vi "Untitled 4.vi"() -> ()   [LabVIEW 2017]
uses:
  <vilib>/Utility/NIReport.llb/Append Text Table to Report (wrap).vi
  <vilib>/Utility/NIReport.llb/NI_report.lvclass
panel:
  in  "Table Control":string[][](table)
  in  "template (empty)":path
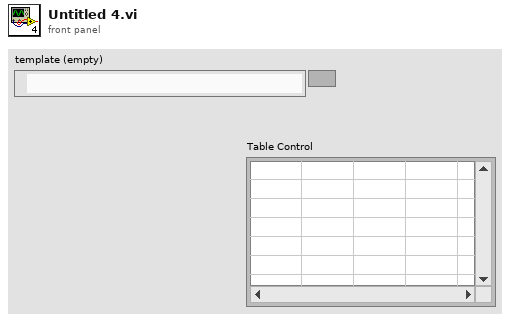
[diagram p1: front panel]
types:
  T1 = cluster{"position (excel)":cluster{"row":i32, "column":i32}, "name (excel)":string, "bookmark (word)":string}
  T2 = enum16{"maximized", "minimized", "normal", "no change"}
  T3 = enum16{"Standard Report", "HTML", "Word", "Excel"}
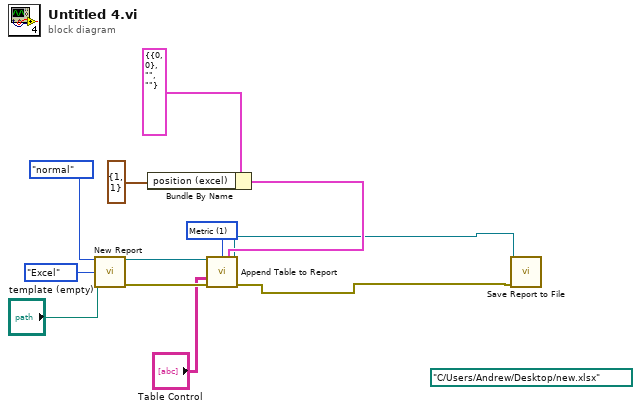
[diagram p0: block diagram]
diagram:
  (unwired) path "C:/Users/Andrew/Desktop/new.xlsx"
  w4 = u16 1 items=["US", "Metric", "Default"] ("measurement system")
  n1 = call <vilib>:"New Report.vi"("window state (normal)"=T2."normal", "report type"=T3."Excel", "template (empty)"="template (empty)") -> ("report out"=w9:refnum<class "NI_report.lvclass">, "error out"=w8:errorcluster)  [unwired: 11 in]
  n2 = Bundle By Name(cluster=T1 {"position (excel)"={"row"=0, "column"=0}, "name (excel)"="", "bookmark (word)"=""} ("MS Office parameters"), "position (excel)"=cluster{"row":i32, "column":i32} {"row"=1, "column"=1}) -> (w5:T1)
  n3 = call-poly <vilib>:"Append Table to Report.vi"("report in"=w9, "measurement system"=w4, "MS Office parameters"=w5, "text data"="Table Control", "error in (no error)"=w8) -> ("report out"=w2:refnum<class "NI_report.lvclass">, "error out"=w1:errorcluster)  [unwired: 7 in, 2 out]
  n4 = call-dynamic "Save Report to File.vi"("report in"=w2, "error in (no error)"=w1) -> ()  [unwired: 12 in, 2 out]
